vi "8.6.-Momento h3.vi"(1 "n30/n12/n21/n03":dbl[](array[numeric])) -> (0 "M3":dbl)   [LabVIEW 2020]
panel:
  # "Visión Artificial - Momentos Invariantes de Hu\nDiego Cervantes Rodríguez\ndicer0.com"
  # "M3 = ((n30-3*n12)^2)+((3*n21-n03)^2)"
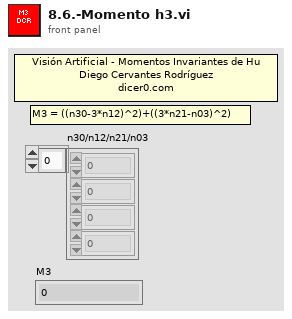
[diagram p1: front panel]
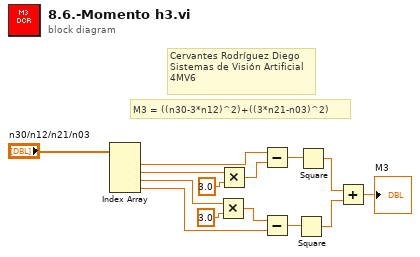
[diagram p0: block diagram]
diagram:
  # "M3 = ((n30-3*n12)^2)+((3*n21-n03)^2)"
  # "Cervantes Rodríguez Diego\nSistemas de Visión Artificial\n4MV6"
  n1 = Index Array "Index Array"(array="n30/n12/n21/n03") -> (element #1=w11:dbl, element #2=w13:dbl, element #3=w9:dbl, element #4=w7:dbl)  [unwired: 4 in]
  n2 = Multiply(x=w9, y=3.0) -> (x*y=w8:dbl)
  n3 = Multiply(x=w13, y=3.0) -> (x*y=w12:dbl)
  n4 = Subtract(x=w11, y=w12) -> (x-y=w10:dbl)
  n5 = Subtract(x=w8, y=w7) -> (x-y=w6:dbl)
  n6 = Square(x=w6) -> (x^2=w4:dbl)
  n7 = Square(x=w10) -> (x^2=w5:dbl)
  n8 = Add(x=w5, y=w4) -> (x+y=→"M3":dbl)
